vi "Check_Dest_Path_Length.vi"(8 "error in (no error)":errorcluster, 10 "file build destinations":string[](array[string]), 11 "Build in":refnum<class "AB_Targetfile.lvclass">) -> (0 "error out":errorcluster, 3 "Build out":refnum<class "AB_Targetfile.lvclass">)   [LabVIEW 2020, in "AB_Targetfile.lvclass"]
uses:
  <vilib>/AppBuilder/AB_Classes/TargetFile/AB_Targetfile.lvclass
  e:/builds/penguin/labview/branches/2020/dev/dist/vi.lib/AppBuilder/AB_Classes/Build/AB_Build.lvclass
  <vilib>/AppBuilder/AB_Classes/Destination/AB_Destination.lvclass
  <vilib>/AppBuilder/AB_Classes/Build/AB_Build.lvclass
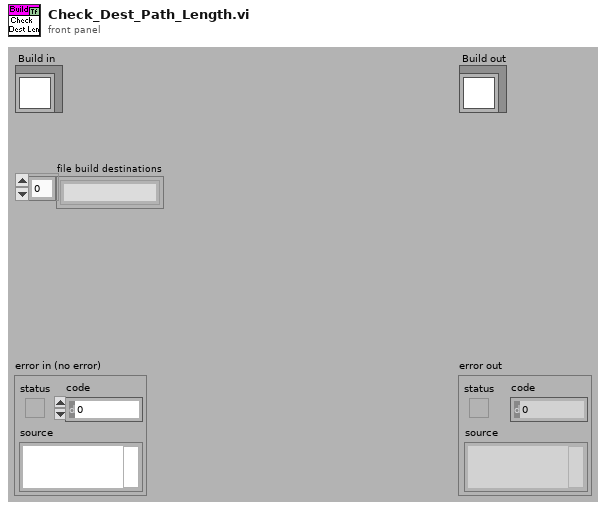
[diagram p1: front panel]
types:
  T1 = typedef "AB_Build.ctl" = cluster{"buildSpecName":string, "buildSpecDescription":string, "destinations":refnum<class "AB_Destination.lvclass">[], "exclusionOption":T2, "defaultLanguage":string, "supportedLanguages":string[], "excludedDirectories":path[], "buildContext":refnum<vi>, "buildObject":T3, "preview":bool, "programatic":bool, "progressBarEvents":T4, "userLog_Path":path, "preActionID":string, "preAction_Path":path, "postActionID":string, "postAction_Path":path, "eng_checkForBrokenVIs?":bool, "eng_verboseLinkerErrors?":bool, "localDest_Path":path, "targetDest_Path":path, "removeVIObject":u16, "cache":refnum<class "PreviewCache.lvclass">, "use cache":bool, "previewCache_ID":string, "buildCache_ID":string, "eng_TempLocalDest_Path":path, "eng_collectDependencies?":bool, "versionInfo":cluster{"buildVersion":cluster{"major":u16, "minor":u16, "patch":u16, "build":u16}, "autoIncrement":bool}, "eng_enableVIChecksums":bool}
  T2 = typedef "AB_Exclusion_Option.ctl" = cluster{"typedefs":bool, "polymorphicVIs":bool, "unusedLibraryItems":bool, "modifyLibraryFile":bool, "edit-timeDependencies":bool, "inlineVIs":bool, "dependent PPLs":bool, "dependent DLLs":bool}
  T3 = typedef "ItemRef.ctl" = u64
  T4 = typedef "provcom_ProgressBar_Events.ctl" = cluster{"newJob":refnum<user-event>, "newItem":refnum<user-event>, "errorMsg":T5, "cancel":refnum<user-event>}
  T5 = typedef "mxLvBuildError.ctl" = refnum<user-event>
  T6 = typedef "AB_Destination.ctl" = cluster{"destName":string, "path":path, "libraryName":string, "preserveHierarchy":bool, "eng_inBuild":bool, "eng_libraryReference":refnum<vi>, "eng_restictAddToNewLibrary":bool}
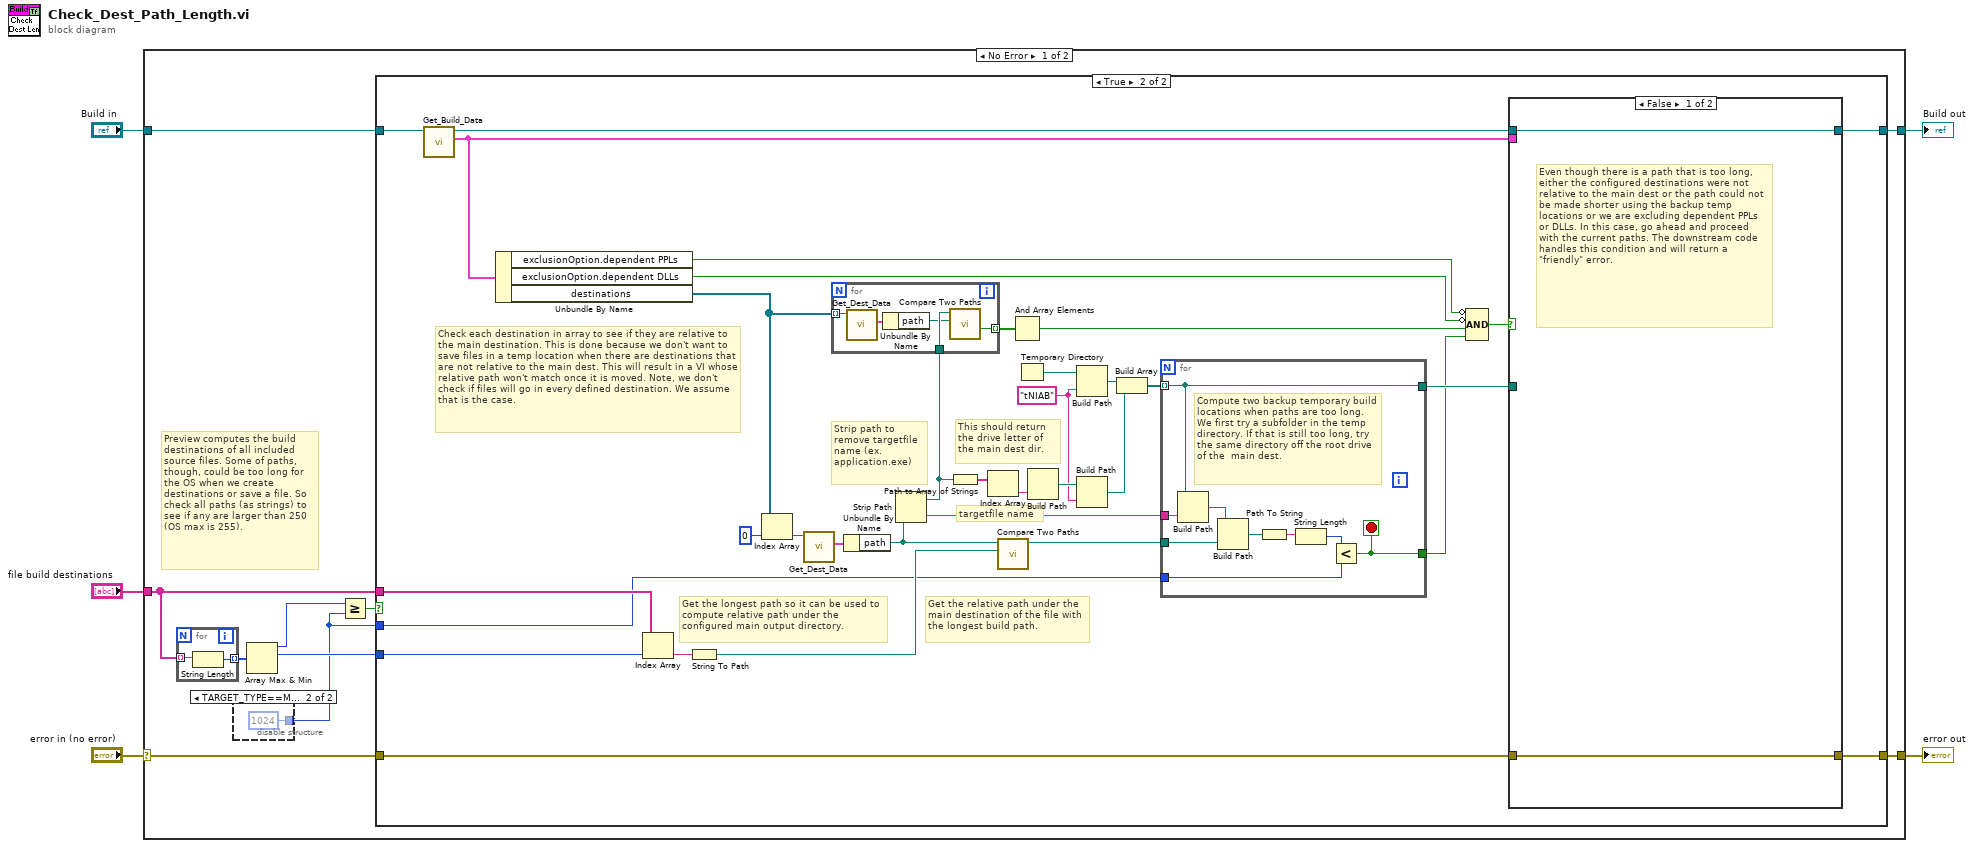
[diagram p0: block diagram]
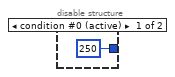
[diagram p2: hidden frame]
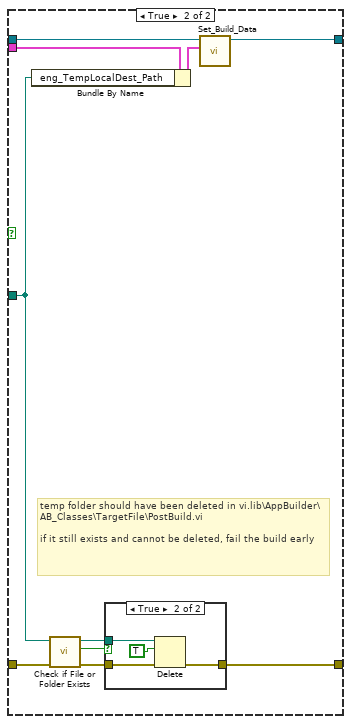
[diagram p4: hidden frame]
diagram:
  n1 = case shown="No Error" "error in (no error)" {
    selector: "error in (no error)" -> [w8 w88]
    tunnel: [w7 w88] -> w1
    tunnel: [w9 w87] -> w5
    tunnel: "Build in" -> [w10 w87]
    tunnel: "file build destinations" -> [w15 _]
    frame No Error {
      # "Preview computes the build destinations of all included source files. Some of paths, though, could be too long for the OS when we create destinations or save a file. So check all paths (as strings) to see if any are larger than 250 (OS max is 255)."
      n2 = for {
        tunnel: w15 -> [w19] mode=indexing
        tunnel: [w18] -> w11 mode=indexing
        n3 = String Length(string=w19) -> (length=w18:i32)
      }
      n4 = disable-structure shown="TARGET_TYPE==Mac" {
        disable-tunnel: [250 ("Maximum Allowable Path Length (252)") 1024 ("Maximum Allowable Path Length (252)")] -> w6
        frame condition #0 (active) {
        }
        frame condition #1 {
        }
      }
      n5 = Array Max & Min(array=w11) -> (max value=w12:i32, max index (indices)=w14:i32)  [unwired: 2 out]
      n6 = Greater Or Equal?(x=w12, y=w6) -> (x >= y?=w13:bool)
      n7 = case shown="True" w13 {
        tunnel: w15 -> [_ w55]
        tunnel: w14 -> [_ w51]
        tunnel: w10 -> [w21 w42]
        tunnel: [w21 w34] -> w9
        tunnel: w6 -> [_ w29]
        tunnel: [w20 w27] -> w7
        tunnel: w8 -> [w20 w28]
        frame False {
          # "If all paths are less than threshold, then proceed with no changes to build destination paths."
        }
        frame True {
          w37 = "tNIAB" ("name or relative path")
          # "Check each destination in array to see if they are relative to the main destination. This is done because we don't want to save files in a temp location when there are destinations that are not relative to the main dest. This will result in a VI whose relative path won't match once it is moved. Note, we don't check if files will go in every defined destination. We assume that is the case."
          # "targetfile name"
          # "Strip path to remove targetfile name (ex. application.exe)"
          # "Get the relative path under the main destination of the file with the longest build path."
          # "This should return the drive letter of the main dest dir."
          # "Get the longest path so it can be used to compute relative path under the configured main output directory."
          n8 = call <vilib>:"Get_Build_Data.vi"("Class in"=w42) -> ("data"=w33:T1, "Class out"=w35:refnum<class "AB_Targetfile.lvclass">)  [unwired: 1 in, 8 out]
          n9 = Unbundle By Name(w33) -> ("exclusionOption.dependent PPLs"=w23:bool, "exclusionOption.dependent DLLs"=w22:bool, "destinations"=w43:refnum<class "AB_Destination.lvclass">[])
          n10 = Index Array(array=w55, index=w51) -> (element=w53:string)
          n11 = String To Path(string=w53) -> (path=w50:path)
          n12 = Index Array(array=w43, index=0) -> (element=w48:refnum<class "AB_Destination.lvclass">)
          n13 = call <vilib>:"Get_Dest_Data.vi"("Class in"=w48) -> ("destName"=w46:T6)  [unwired: 8 in, 2 out]
          n14 = Unbundle By Name(w46) -> ("path"=w45:path)
          n15 = Strip Path(path=w45) -> (stripped path=w39:path, name=w44:string)
          n16 = for {
            tunnel: w43 -> [w68] mode=indexing
            tunnel: w39 -> [w66]
            tunnel: [w67] -> w49 mode=indexing
            n17 = call <vilib>:"Get_Dest_Data.vi"("Class in"=w68) -> ("destName"=w69:T6)  [unwired: 8 in, 2 out]
            n18 = Unbundle By Name(w69) -> ("path"=w65:path)
            n19 = call <vilib>:"Compare Two Paths.vi"("Path 2"=w65, "Path 1"=w66) -> ("Path 2 Relative to Path 1?"=w67:bool)  [unwired: 6 in, 3 out]
          }
          n20 = Path to Array of Strings(0:w39) -> (2:w41:string[])  [unwired: 1 out]
          n21 = Index Array(array=w41) -> (element=w40:string)  [unwired: 1 in]
          n22 = call <vilib>:"Compare Two Paths.vi"("Path 2"=w50, "Path 1"=w45) -> ("Relative Path from 1 to 2"=w54:path)  [unwired: 6 in, 3 out]
          n23 = And Array Elements(Boolean array=w49) -> (logical AND=w26:bool)
          n24 = Temporary Directory() -> (w52:path)
          n25 = Build Path(name or relative path=w40) -> (appended path=w38:path)  [unwired: 1 in]
          n26 = Build Path(base path=w52, name or relative path=w37) -> (appended path=w32:path)
          n27 = Build Path(base path=w38, name or relative path=w37) -> (appended path=w31:path)
          n28 = Build Array(w32, w31) -> (w36:path[])
          n29 = for {
            tunnel: w54 -> [w63]
            tunnel: [w58] -> w25
            tunnel: w44 -> [w59]
            tunnel: w36 -> [w57] mode=indexing
            tunnel: [w57] -> w30
            tunnel: w29 -> [w56]
            stop <- w58 stop-if-true
            # "Compute two backup temporary build locations when paths are too long. We first try a subfolder in the temp directory. If that is still too long, try the same directory off the root drive of the  main dest."
            n30 = Build Path(base path=w57, name or relative path=w59) -> (appended path=w60:path)
            n31 = Build Path(base path=w60, name or relative path=w63) -> (appended path=w62:path)
            n32 = Path To String(path=w62) -> (string=w64:string)
            n33 = String Length(string=w64) -> (length=w61:i32)
            n34 = Less?(x=w61, y=w56) -> (x < y?=w58:bool)
          }
          n35 = Compound Arithmetic op=AND(invert w23, invert w22, w26, w25) -> (w24:bool)
          n36 = case shown="False" w24 {
            tunnel: w35 -> [w71 w81]
            tunnel: [w71 w80] -> w34
            tunnel: w33 -> [_ w79]
            tunnel: w30 -> [_ w74]
            tunnel: w28 -> [w70 w76]
            tunnel: [w70 w77] -> w27
            frame False {
              # "Even though there is a path that is too long, either the configured destinations were not relative to the main dest or the path could not be made shorter using the backup temp locations or we are excluding dependent PPLs or DLLs. In this case, go ahead and proceed with the current paths. The downstream code handles this condition and will return a \"friendly\" error."
            }
            frame True {
              # "temp folder should have been deleted in vi.lib\\AppBuilder\\AB_Classes\\TargetFile\\PostBuild.vi\n\nif it still exists and cannot be deleted, fail the build early"
              n37 = Bundle By Name(cluster=w79, "eng_TempLocalDest_Path"=w74) -> (w78:T1)
              n38 = call <vilib>:"Check if File or Folder Exists.vi"("error in (no error)"=w76, "path"=w74) -> ("error out"=w75:errorcluster, "file or folder exists?"=w72:bool, "dup path"=w73:path)  [unwired: 7 in]
              n39 = case shown="True" w72 {
                tunnel: [w82 w85] -> w77
                tunnel: w75 -> [w82 w84]
                tunnel: w73 -> [_ w83]
                frame False {
                }
                frame True {
                  n40 = Delete(path (use dialog)=w83, entire hierarchy (F)=TRUE, error in=w84) -> (error out=w85:errorcluster)  [unwired: 4 out]
                }
              }
              n41 = call <vilib>:"Set_Build_Data.vi"("data"=w78, "Class in"=w81) -> ("Class out"=w80:refnum<class "AB_Targetfile.lvclass">)  [unwired: 8 in, 1 out]
            }
          }
        }
      }
    }
    frame Error {
    }
  }
  "error out" <- w1
  "Build out" <- w5
